vi "FillString.vi"(8 "error in":errorcluster caption="错误输入（无错误）", 9 "PackLen":u32, 10 "Fill?":bool=TRUE, 11 "StringIn":string) -> (0 "error out":errorcluster caption="错误输出", 3 "StringOut":string)   [LabVIEW 2013]
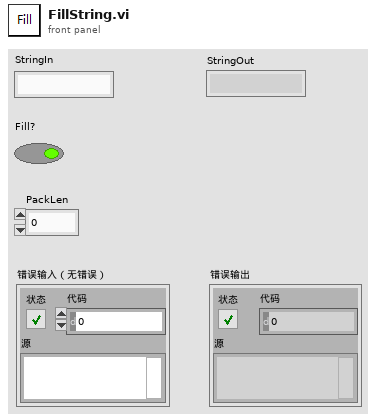
[diagram p1: front panel]
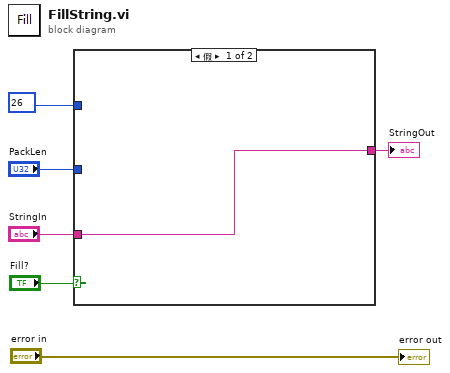
[diagram p0: block diagram]
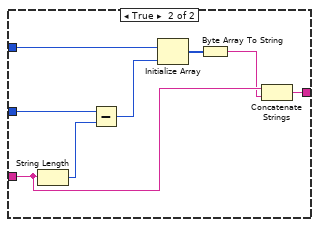
[diagram p2: hidden frame]
diagram:
  n1 = case shown="假" "Fill?" {
    tunnel: "PackLen" -> [_ w15]
    tunnel: u8 26 -> [_ w13]
    tunnel: "StringIn" -> [w7 w10]
    tunnel: [w7 w8] -> w3
    frame False {
    }
    frame True {
      n2 = String Length(string=w10) -> (length=w14:i32)
      n3 = Subtract(x=w15, y=w14) -> (x-y=w12:u32)
      n4 = Initialize Array(w13, w12) -> (w11:u8[])
      n5 = Byte Array To String(unsigned byte array=w11) -> (string=w9:string)
      n6 = Concatenate Strings(w10, w9) -> (w8:string)
    }
  }
  "StringOut" <- w3
  "error out" <- "error in"
